vi "Client Connection State Callback.vi"(7 "Owner":refnum<class>, 8 "error in (no error)":errorcluster, 9 "Variant":variant, 10 "Connection State":T1, 11 "Connection":refnum<class "Connection.lvclass">) -> (0 "error out":errorcluster)   [LabVIEW 2020, in "TCP Tests.lvlib"]
uses:
  TCP Tests.lvlib
  lv-stream/stream/Connection/Connection.lvclass
  C:/Program Files (x86)/National Instruments/LabVIEW 2020/vi.lib/IlluminatedG/lv-stream/Endpoint/Endpoint.lvclass
  lv-stream/stream/Connection State.ctl
  lv-stream/stream/Endpoint/Endpoint.lvclass
  lv-stream/stream/Stream.lvlib
panel:
  out "Reconnects":i32
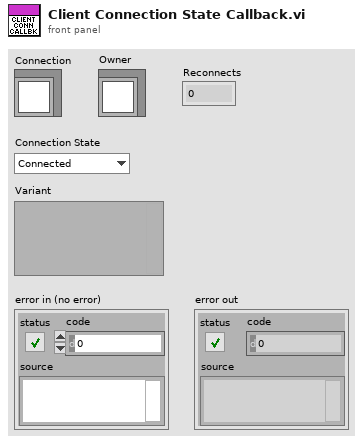
[diagram p1: front panel]
types:
  T1 = typedef "Stream.lvlib/Connection State.ctl" = enum16{"Connected", "Disconnected"}
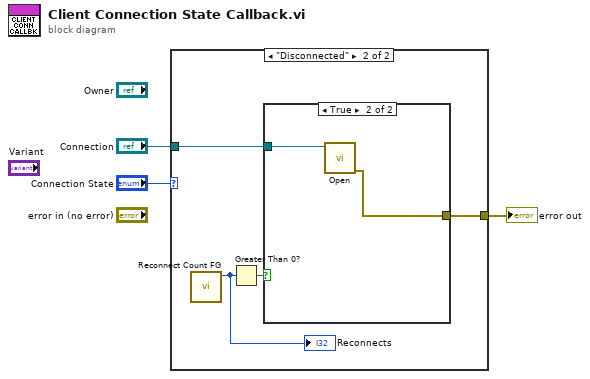
[diagram p0: block diagram]
diagram:
  n1 = case shown="\"Disconnected\"" "Connection State" {
    tunnel: "Connection" -> [_ w7]
    tunnel: [_ w4] -> w1
    frame "Connected" {
    }
    frame "Disconnected" {
      n2 = call "Reconnect Count FG.vi"() -> ("s? t:f"=w5:i32)  [unwired: 11 in]
      "Reconnects" <- w5
      n3 = Greater Than 0?(x=w5) -> (x > 0?=w6:bool)
      n4 = case shown="True" w6 {
        tunnel: w7 -> [_ w9]
        tunnel: [_ w8] -> w4
        frame False {
        }
        frame True {
          n5 = call "Open.vi"("Endpoint in"=w9) -> ("error out"=w8:errorcluster)  [unwired: 9 in, 1 out]
        }
      }
    }
  }
  "error out" <- w1
